vi "Get Caption - Add To Owner.vi"(1 "Owner Filename (incl. file extension)":string) -> (0 "\"Add To Owner\" caption":string)   [LabVIEW 2022 SP3]
doc: "<add documentation here>"
panel:
  # "Development\nControls or indicators that are useful for development or testing, but which are not outputs of the VI."
  # "Input\nInputs to the VI"
  # "Output\nOutputs of the VI"
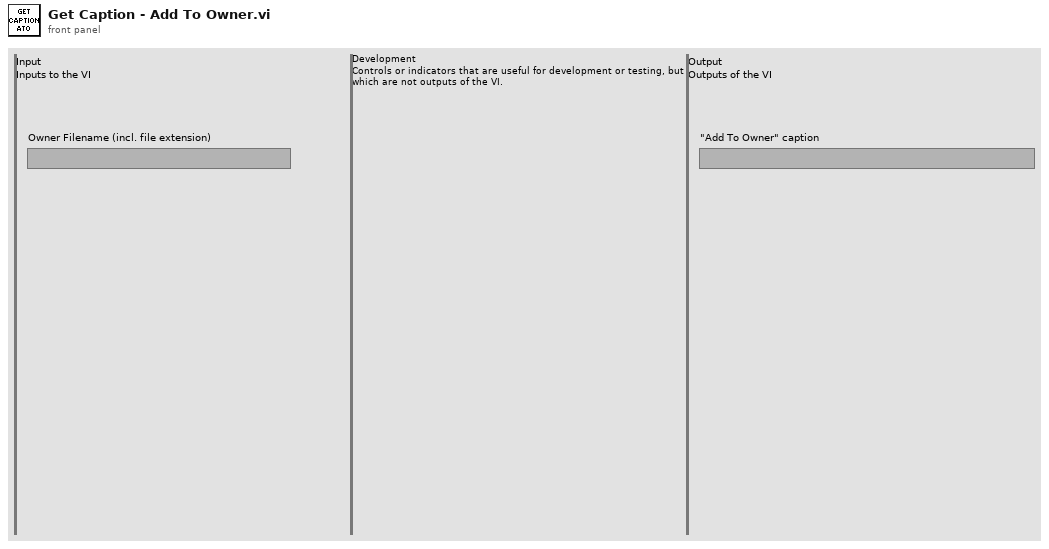
[diagram p1: front panel]
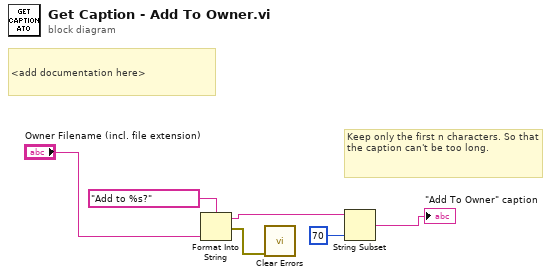
[diagram p0: block diagram]
diagram:
  # "Keep only the first n characters. So that the caption can't be too long."
  # "<add documentation here>"
  n1 = Format Into String(format string="Add to %s?" ("Caption.Text"), "Owner Filename (incl. file extension)") -> (resulting string=w4:string, error out=w5:errorcluster)  [unwired: 2 in]
  n2 = call <vilib>:"Clear Errors.vi"("error in (no error)"=w5) -> ()  [unwired: 5 in, 2 out]
  n3 = String Subset(string=w4, length (rest)=70 ("length (rest)")) -> (substring=→"\"Add To Owner\" caption":string)  [unwired: 1 in]
